vi "RichToFlatniswitch_grpc_RouteTriggerInputRequest.vi"(5 "OutputClusterType":T1, 11 "InputCluster":T4) -> (3 "OutputCluster":T1)   [LabVIEW 2021, in "NI Switch_client.lvlib"]
uses:
  NI Switch_client.lvlib
  niswitch_grpc_RouteTriggerInputRequest.ctl
  niswitch_grpc_RouteTriggerInputRequest_trigger_input_connector_enum/niswitch_grpc_RouteTriggerInputRequest_trigger_input_connector_enum.lvclass
  niswitch_grpc_RouteTriggerInputRequest_trigger_input_bus_line_enum/niswitch_grpc_RouteTriggerInputRequest_trigger_input_bus_line_enum.lvclass
  nidevice_grpc_Session.ctl
  niswitch_grpc_RouteTriggerInputRequest_Flat.ctl
  nidevice_grpc_Session_Flat.ctl
  niswitch_grpc_TriggerInput.ctl
  niswitch_grpc_RouteTriggerInputRequest_trigger_input_connector_enum/niswitch_grpc_RouteTriggerInputRequest_trigger_input_connector_enum.lvclass/niswitch_grpc_RouteTriggerInputRequest_trigger_input_connector_enum.ctl
  niswitch_grpc_RouteTriggerInputRequest_trigger_input_bus_line_enum/niswitch_grpc_RouteTriggerInputRequest_trigger_input_bus_line_enum.lvclass/niswitch_grpc_RouteTriggerInputRequest_trigger_input_bus_line_enum.ctl
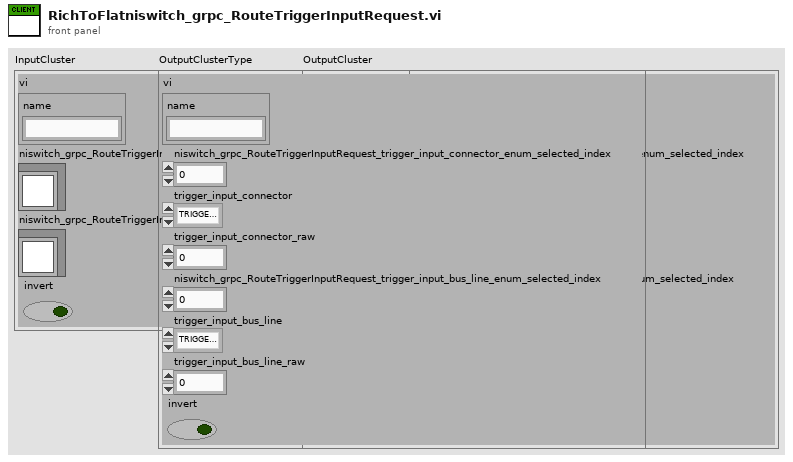
[diagram p1: front panel]
types:
  T1 = typedef "NI Switch_client.lvlib/niswitch_grpc_RouteTriggerInputRequest_Flat.ctl" = cluster{"vi":T2, "niswitch_grpc_RouteTriggerInputRequest_trigger_input_connector_enum_selected_index":i32, "trigger_input_connector":T3, "trigger_input_connector_raw":i32, "niswitch_grpc_RouteTriggerInputRequest_trigger_input_bus_line_enum_selected_index":i32, "trigger_input_bus_line":T3, "trigger_input_bus_line_raw":i32, "invert":bool}
  T2 = typedef "NI Switch_client.lvlib/nidevice_grpc_Session_Flat.ctl" = cluster{"name":string}
  T3 = typedef "NI Switch_client.lvlib/niswitch_grpc_TriggerInput.ctl" = enum32{"TRIGGER_INPUT_UNSPECIFIED", "TRIGGER_INPUT_NISWITCH_VAL_IMMEDIATE", "TRIGGER_INPUT_NISWITCH_VAL_EXTERNAL", "TRIGGER_INPUT_NISWITCH_VAL_SOFTWARE_TRIG", "TRIGGER_INPUT_NISWITCH_VAL_TTL0", "TRIGGER_INPUT_NISWITCH_VAL_TTL1", "TRIGGER_INPUT_NISWITCH_VAL_TTL2", "TRIGGER_INPUT_NISWITCH_VAL_TTL3", "TRIGGER_INPUT_NISWITCH_VAL_TTL4", "TRIGGER_INPUT_NISWITCH_VAL_TTL5", "TRIGGER_INPUT_NISWITCH_VAL_TTL6", "TRIGGER_INPUT_NISWITCH_VAL_TTL7", "TRIGGER_INPUT_NISWITCH_VAL_PXI_STAR", "TRIGGER_INPUT_NISWITCH_VAL_REARCONNECTOR", "TRIGGER_INPUT_NISWITCH_VAL_FRONTCONNECTOR", "TRIGGER_INPUT_NISWITCH_VAL_REARCONNECTOR_MODULE1", "TRIGGER_INPUT_NISWITCH_VAL_REARCONNECTOR_MODULE2", "TRIGGER_INPUT_NISWITCH_VAL_REARCONNECTOR_MODULE3", "TRIGGER_INPUT_NISWITCH_VAL_REARCONNECTOR_MODULE4", "TRIGGER_INPUT_NISWITCH_VAL_REARCONNECTOR_MODULE5", "TRIGGER_INPUT_NISWITCH_VAL_REARCONNECTOR_MODULE6", "TRIGGER_INPUT_NISWITCH_VAL_REARCONNECTOR_MODULE7", "TRIGGER_INPUT_NISWITCH_VAL_REARCONNECTOR_MODULE8", "TRIGGER_INPUT_NISWITCH_VAL_REARCONNECTOR_MODULE9", "TRIGGER_INPUT_NISWITCH_VAL_REARCONNECTOR_MODULE10", "TRIGGER_INPUT_NISWITCH_VAL_REARCONNECTOR_MODULE11", "TRIGGER_INPUT_NISWITCH_VAL_REARCONNECTOR_MODULE12", "TRIGGER_INPUT_NISWITCH_VAL_FRONTCONNECTOR_MODULE1", "TRIGGER_INPUT_NISWITCH_VAL_FRONTCONNECTOR_MODULE2", "TRIGGER_INPUT_NISWITCH_VAL_FRONTCONNECTOR_MODULE3", "TRIGGER_INPUT_NISWITCH_VAL_FRONTCONNECTOR_MODULE4", "TRIGGER_INPUT_NISWITCH_VAL_FRONTCONNECTOR_MODULE5", "TRIGGER_INPUT_NISWITCH_VAL_FRONTCONNECTOR_MODULE6", "TRIGGER_INPUT_NISWITCH_VAL_FRONTCONNECTOR_MODULE7", "TRIGGER_INPUT_NISWITCH_VAL_FRONTCONNECTOR_MODULE8", "TRIGGER_INPUT_NISWITCH_VAL_FRONTCONNECTOR_MODULE9", "TRIGGER_INPUT_NISWITCH_VAL_FRONTCONNECTOR_MODULE10", "TRIGGER_INPUT_NISWITCH_VAL_FRONTCONNECTOR_MODULE11", "TRIGGER_INPUT_NISWITCH_VAL_FRONTCONNECTOR_MODULE12"}
  T4 = typedef "NI Switch_client.lvlib/niswitch_grpc_RouteTriggerInputRequest.ctl" = cluster{"vi":T5, "niswitch_grpc_RouteTriggerInputRequest_trigger_input_connector_enum":refnum<class "niswitch_grpc_RouteTriggerInputRequest_trigger_input_connector_enum.lvclass">, "niswitch_grpc_RouteTriggerInputRequest_trigger_input_bus_line_enum":refnum<class "niswitch_grpc_RouteTriggerInputRequest_trigger_input_bus_line_enum.lvclass">, "invert":bool}
  T5 = typedef "NI Switch_client.lvlib/nidevice_grpc_Session.ctl" = cluster{"name":string}
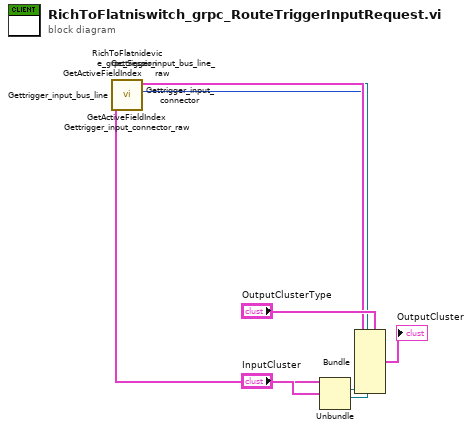
[diagram p0: block diagram]
diagram:
  n1 = Unbundle "Unbundle"("InputCluster") -> ("vi"=w11:T5, "niswitch_grpc_RouteTriggerInputRequest_trigger_input_connector_enum"=w9:refnum<class "niswitch_grpc_RouteTriggerInputRequest_trigger_input_connector_enum.lvclass">, "niswitch_grpc_RouteTriggerInputRequest_trigger_input_bus_line_enum"=w5:refnum<class "niswitch_grpc_RouteTriggerInputRequest_trigger_input_bus_line_enum.lvclass">, "invert"=w1:bool)
  n2 = call "Gettrigger_input_bus_line_raw.vi"("OneOfTemplate in"=w5) -> ("Get_Val"=w2:i32)  [unwired: 8 in, 2 out]
  n3 = call "Gettrigger_input_bus_line.vi"("OneOfTemplate in"=w5) -> ("Get_Val"=w3:T3)  [unwired: 8 in, 2 out]
  n4 = call "GetActiveFieldIndex.vi"("OneOfTemplate in"=w5) -> ("Active Field Index"=w4:i32)  [unwired: 8 in, 2 out]
  n5 = call "Gettrigger_input_connector_raw.vi"("OneOfTemplate in"=w9) -> ("Get_Val"=w6:i32)  [unwired: 8 in, 2 out]
  n6 = call "Gettrigger_input_connector.vi"("OneOfTemplate in"=w9) -> ("Get_Val"=w7:T3)  [unwired: 8 in, 2 out]
  n7 = call "GetActiveFieldIndex.vi"("OneOfTemplate in"=w9) -> ("Active Field Index"=w8:i32)  [unwired: 8 in, 2 out]
  n8 = call "RichToFlatnidevice_grpc_Session.vi"("InputCluster"=w11) -> ("OutputCluster"=w10:T2)  [unwired: 10 in]
  n9 = Bundle "Bundle"(cluster="OutputClusterType", "vi"=w10, "niswitch_grpc_RouteTriggerInputRequest_trigger_input_connector_enum_selected_index"=w8, "trigger_input_connector"=w7, "trigger_input_connector_raw"=w6, "niswitch_grpc_RouteTriggerInputRequest_trigger_input_bus_line_enum_selected_index"=w4, "trigger_input_bus_line"=w3, "trigger_input_bus_line_raw"=w2, "invert"=w1) -> (→"OutputCluster":T1)
